vi "TriggerCollection.vi"(6 "rules":T1[](array[typedef]), 8 "error in (no error)":errorcluster, 9 "collect file":bool, 10 "updates":T5[](array[typedef]), 11 "map":T7) -> (0 "error out":errorcluster)   [LabVIEW 2017, in "TrendAlarm.lvlib"]
uses:
  <vilib>/addons/InsightCM/Devices/Shared/Common/TrendAlarm/TrendAlarm.lvlib
  <vilib>/addons/PointValueMap/controls/PointMap.ctl
  <vilib>/addons/InsightCM/Devices/Shared/Common/TrendAlarm/controls/TransitionCache.ctl
  <vilib>/addons/InsightCM/MessageBus/Base/controls/TrendAlarmTransition.ctl
  <vilib>/addons/InsightCM/MessageBus/Base/controls/TrendAlarmRule.ctl
  <vilib>/addons/InsightCM/MessageBus/Base/controls/TrendAlarmLevel.ctl
  <vilib>/addons/InsightCM/MessageBus/Base/controls/AlarmAction.ctl
  <vilib>/addons/InsightCM/MessageBus/Base/controls/KeyValuePair.ctl
  <vilib>/addons/InsightCM/Devices/Shared/Common/DataEventCreator/controls/Reason.ctl
  <vilib>/addons/InsightCM/MessageBus/Base/controls/TrendAlarmUpdate.ctl
  <vilib>/addons/PointValueMap/subVIs/Point_Write_variant.vi
  <vilib>/addons/PointValueMap/subVIs/Point_Write_string.vi
  <vilib>/addons/PointValueMap/subVIs/Point_Write_i32.vi
  <vilib>/addons/PointValueMap/PointValueMap.lvlib
  <vilib>/addons/InsightCM/Devices/Shared/Common/DataEventCreator/DataEventCreator.lvlib
  <vilib>/addons/InsightCM/Utilities/PropertyHelpers/PropertyHelpers.lvlib
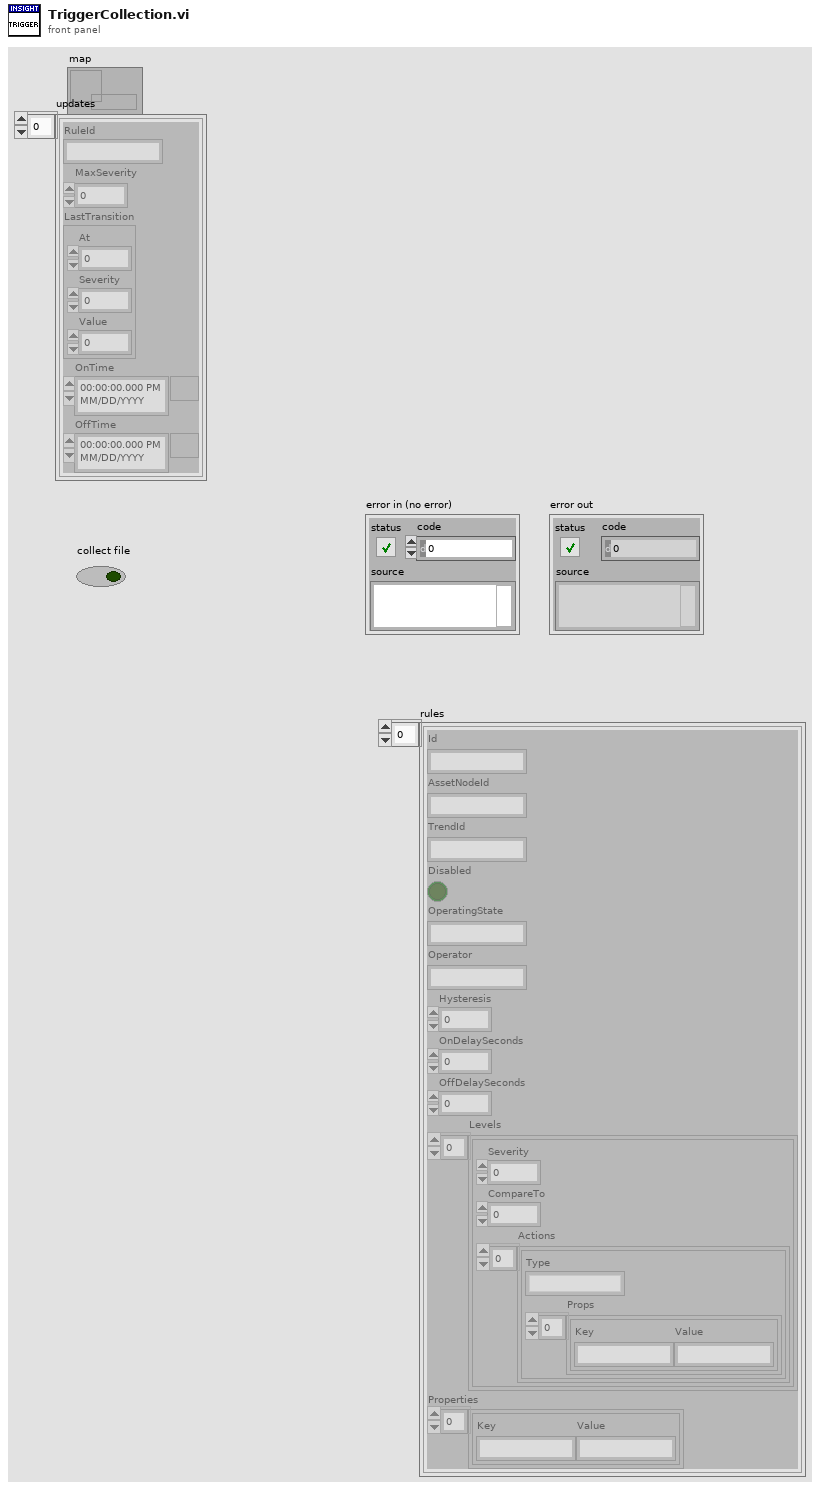
[diagram p1: front panel]
types:
  T1 = typedef "TrendAlarmRule.ctl" = cluster{"Id":string, "AssetNodeId":string, "TrendId":string, "Disabled":bool, "OperatingState":string, "Operator":string, "Hysteresis":dbl, "OnDelaySeconds":dbl, "OffDelaySeconds":dbl, "Levels":T2[], "Properties":T4[]}
  T2 = typedef "TrendAlarmLevel.ctl" = cluster{"Severity":i32, "CompareTo":dbl, "Actions":T3[]}
  T3 = typedef "AlarmAction.ctl" = cluster{"Type":string, "Props":T4[]}
  T4 = typedef "KeyValuePair.ctl" = cluster{"Key":string, "Value":string}
  T5 = typedef "TrendAlarm.lvlib/TransitionCache.ctl" = cluster{"RuleId":string, "MaxSeverity":i32, "LastTransition":T6, "OnTime":timestamp, "OffTime":timestamp}
  T6 = typedef "TrendAlarmTransition.ctl" = cluster{"At":i64, "Severity":i32, "Value":dbl}
  T7 = typedef "PointValueMap.lvlib/PointMap.ctl" = refnum<data-value>
  T8 = typedef "DataEventCreator.lvlib/Reason.ctl" = enum16{"Periodic Event", "Delta EU Event", "Trend Event", "Alarm Event", "User Event", "Enter Operating State", "Exit Operating State", "Multiple Events", "Other"}
  T9 = typedef "TrendAlarmUpdate.ctl" = cluster{"RuleId":string, "Transition":T6}
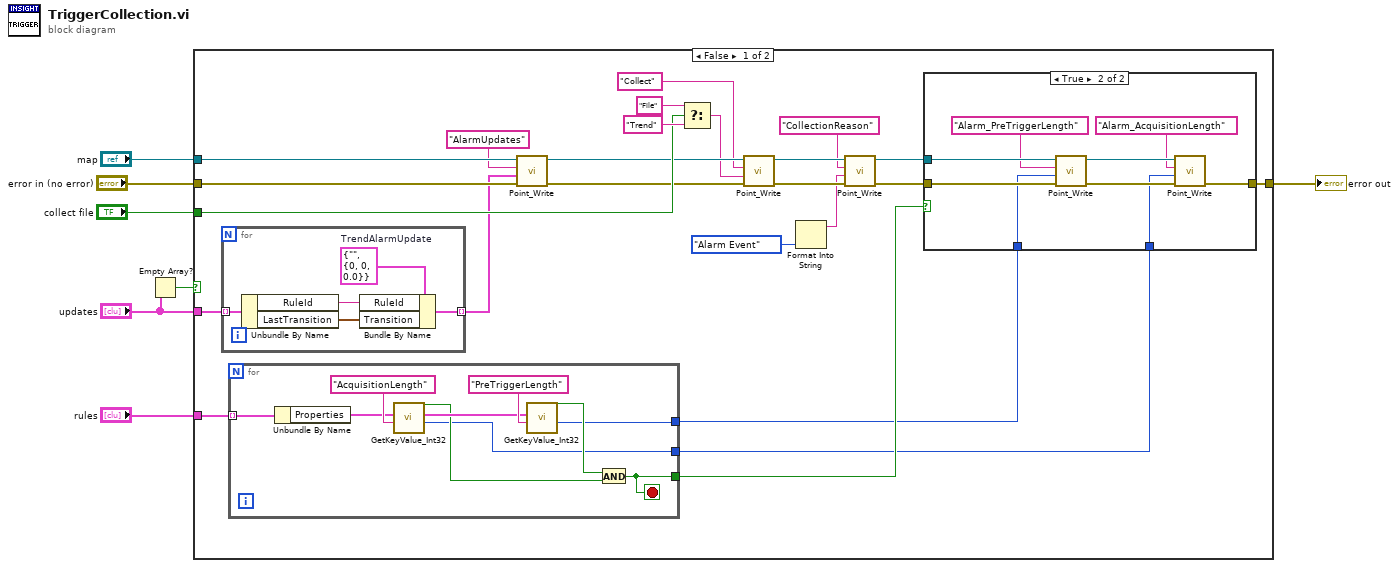
[diagram p0: block diagram]
diagram:
  n1 = Empty Array?(array="updates") -> (empty?=w6:bool)
  n2 = case shown="False" w6 {
    tunnel: "error in (no error)" -> [w24 w57]
    tunnel: [w11 w57] -> w4
    tunnel: "map" -> [w26 _]
    tunnel: "collect file" -> [w27 _]
    tunnel: "updates" -> [w21 _]
    tunnel: "rules" -> [w14 _]
    frame False {
      n3 = for {
        tunnel: w21 -> [w56] mode=indexing
        tunnel: [w52] -> w20 mode=indexing
        w55 = T9 {"RuleId"="", "Transition"={"At"=0, "Severity"=0, "Value"=0.0}}  # TrendAlarmUpdate
        n4 = Unbundle By Name(w56) -> ("RuleId"=w54:string, "LastTransition"=w53:T6)
        n5 = Bundle By Name(cluster=w55, "RuleId"=w54, "Transition"=w53) -> (w52:T9)
      }
      n6 = for {
        tunnel: w14 -> [w49] mode=indexing
        tunnel: [w44] -> w8
        tunnel: [w43] -> w9
        tunnel: [w42] -> w10
        stop <- w42 stop-if-true
        n7 = Unbundle By Name(w49) -> ("Properties"=w50:T4[])
        n8 = call <vilib>:"GetKeyValue_Int32.vi"("key"="AcquisitionLength", "key value pairs"=w50) -> ("value"=w44:i32, "key value pairs out"=w47:T4[], "found"=w45:bool)  [unwired: 7 in]
        n9 = call <vilib>:"GetKeyValue_Int32.vi"("key"="PreTriggerLength", "key value pairs"=w47) -> ("value"=w43:i32, "found"=w46:bool)  [unwired: 7 in, 1 out]
        n10 = And(x=w46, y=w45) -> (x .and. y?=w42:bool)
      }
      n11 = call-poly <vilib>:"Point_Write.vi"("Error In"=w24, "Value"=w20, "Tag"="AlarmUpdates", "Map"=w26) -> ("Error Out"=w23:errorcluster, "Map Out"=w25:T7)  [unwired: 6 in]
      n12 = Select(t="File" ("Tag"), s=w27, f="Trend" ("Tag")) -> (s? t:f=w19:string)
      n13 = call-poly <vilib>:"Point_Write.vi"("Error In"=w23, "Value"=w19, "Tag"="Collect", "Map"=w25) -> ("Error Out"=w31:errorcluster, "Map Out"=w30:T7)  [unwired: 6 in]
      n14 = Format Into String(Reason."Alarm Event" ("Reason")) -> (resulting string=w15:string)  [unwired: 3 in, 1 out]
      n15 = call-poly <vilib>:"Point_Write.vi"("Error In"=w31, "Value"=w15, "Tag"="CollectionReason", "Map"=w30) -> ("Error Out"=w12:errorcluster, "Map Out"=w13:T7)  [unwired: 6 in]
      n16 = case shown="True" w10 {
        tunnel: w13 -> [_ w41]
        tunnel: w12 -> [w32 w37]
        tunnel: [w32 w35] -> w11
        tunnel: w9 -> [_ w34]
        tunnel: w8 -> [_ w33]
        frame False {
        }
        frame True {
          n17 = call-poly <vilib>:"Point_Write.vi"("Error In"=w37, "Value"=w34, "Tag"="Alarm_PreTriggerLength", "Map"=w41) -> ("Error Out"=w36:errorcluster, "Map Out"=w40:T7)  [unwired: 6 in]
          n18 = call-poly <vilib>:"Point_Write.vi"("Error In"=w36, "Value"=w33, "Tag"="Alarm_AcquisitionLength", "Map"=w40) -> ("Error Out"=w35:errorcluster)  [unwired: 6 in, 1 out]
        }
      }
    }
    frame True {
    }
  }
  "error out" <- w4
